vi "About Dialog.vi"(8 "error in (no error)":errorcluster) -> (0 "error out":errorcluster)   [LabVIEW 2019]
doc: "Open About Dialog."
panel:
  out "Titel":string
  out "Version Info":string
  out "License Code":string
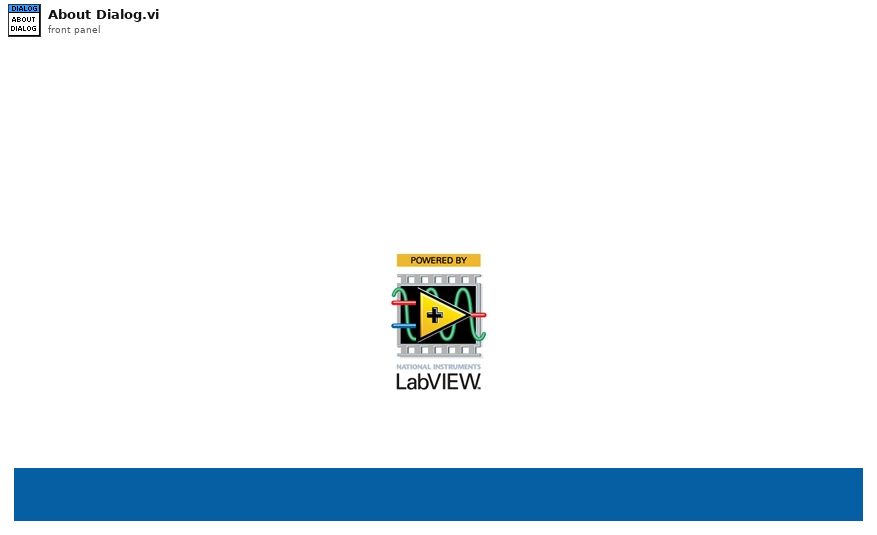
[diagram p1: front panel]
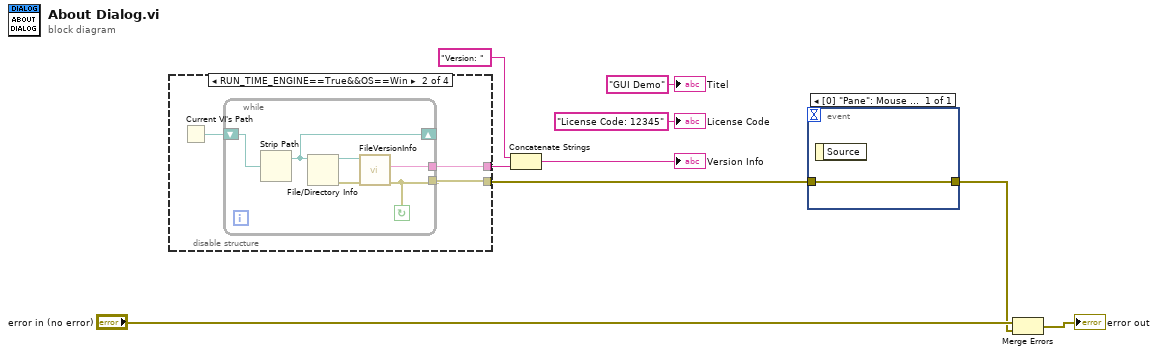
[diagram p0: block diagram]
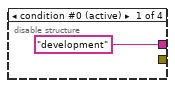
[diagram p2: hidden frame]
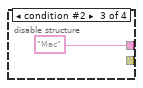
[diagram p3: hidden frame]
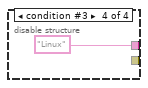
[diagram p4: hidden frame]
diagram:
  n1 = disable-structure "Conditional Disable Structure" shown="RUN_TIME_ENGINE==True&&OS==Win" {
    disable-tunnel: ["development" w13 "Mac" "Linux"] -> w5
    disable-tunnel: [_ w12 _ _] -> w2
    frame condition #0 (active) {
    }
    frame condition #1 {
      n2 = Current VI's Path() -> (path=w11:path)
      n3 = while {
        tunnel: [w17] -> w13
        tunnel: [w16] -> w12
        shift-right: [w14] -> _
        shift-left: w11 -> [w15]
        stop <- w16 continue-if-true
        n4 = Strip Path(path=w15) -> (stripped path=w14:path)  [unwired: 1 out]
        n5 = File/Directory Info(path=w14) -> (path out=w18:path, error out=w19:errorcluster)  [unwired: 1 in, 5 out]
        n6 = call <vilib>:"FileVersionInfo.vi"("error in (no error)"=w19, "Application Path in"=w18) -> ("error out"=w16:errorcluster, "File Version Info"=w17:string)  [unwired: 6 in, 2 out]
      }
    }
    frame condition #2 {
    }
    frame condition #3 {
    }
  }
  n7 = Concatenate Strings("Version: " ("Version Info"), w5) -> (→"Version Info":string)
  n8 = event shown="[0] \"Pane\": Mouse Down" {
    selector: _ -> [_]
    dyn-events: _ -> [_]
    timeout: _ -> [_]
    tunnel: w2 -> [w22]
    tunnel: [w22] -> w1
    event Mouse Down {
      n9 = event-data() -> ()  [unwired: 1 in, 1 out]
    }
  }
  n10 = Merge Errors("error in (no error)", w1) -> (→"error out":errorcluster)
  "Titel" <- "GUI Demo" ("Titel")
  "License Code" <- "License Code: 12345" ("License Code")
